vi "Keyence.Cmd.Save.vi"(6 "Timeout [ms] (1000)":i32=1000, 8 "error in":errorcluster, 11 "cID in":refnum<k5>) -> (0 "error out":errorcluster, 1 "OK?":bool, 3 "cID out":refnum<k5>)   [LabVIEW 2016]
panel:
  out "Response":string
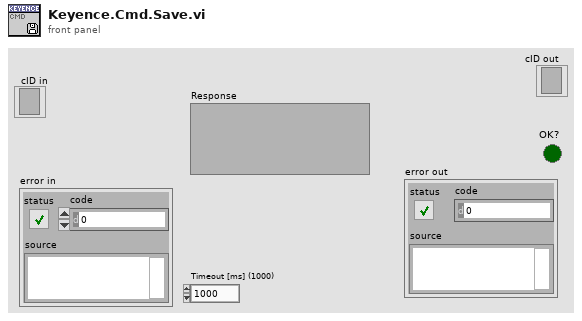
[diagram p1: front panel]
types:
  T1 = enum16{"Standard", "Buffered", "CRLF", "Immediate"}
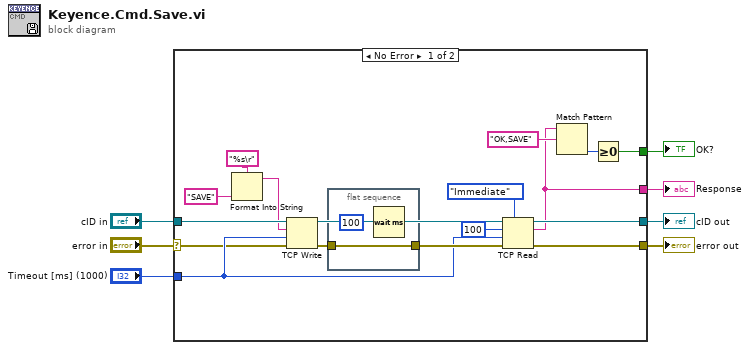
[diagram p0: block diagram]
diagram:
  n1 = case shown="No Error" "error in" {
    selector: "error in" -> [w19 w27]
    tunnel: "Timeout [ms] (1000)" -> [w21 _]
    tunnel: "cID in" -> [w20 w28]
    tunnel: [w13 w28] -> w4
    tunnel: [w14 w27] -> w3
    tunnel: [w12 _] -> w2
    tunnel: [w11 _] -> w1
    frame No Error {
      n2 = Format Into String(format string="%s\r" ("data in"), "SAVE" ("data in")) -> (resulting string=w8:string)  [unwired: 2 in, 1 out]
      n3 = TCP Write(connection ID=w20, data in=w8, error in (no error)=w19, 9:w21) -> (connection ID out=w22:refnum<k5>, error out=w24:errorcluster)  [unwired: 1 out]
      n4 = flat-sequence {
        tunnel: w24 -> [w26]
        tunnel: [w26] -> w23
        frame #0 {
          n5 = Wait (ms)(milliseconds to wait=u32 100) -> ()  [unwired: 1 out]
        }
      }
      n6 = TCP Read(connection ID=w22, bytes to read=100, error in (no error)=w23, 7:T1."Immediate" ("mode (standard)"), 9:w21) -> (connection ID out=w13:refnum<k5>, data out=w11:string, error out=w14:errorcluster)
      n7 = Match Pattern(string=w11, regular expression="OK,SAVE") -> (offset past match=w15:i32)  [unwired: 1 in, 3 out]
      n8 = Greater Or Equal To 0?(x=w15) -> (x >= 0?=w12:bool)
    }
    frame Error {
    }
  }
  "cID out" <- w4
  "Response" <- w1
  "OK?" <- w2
  "error out" <- w3
